vi "To Angle.vi"(1 "Reset":bool, 2 "Tolerance":dbl=1.0 format="%#_13g", 3 "Min. Power":dbl=0.1 format="%#_13g", 4 "Destination Angle":dbl) -> (0 "Power Change":dbl)   [LabVIEW 2014]
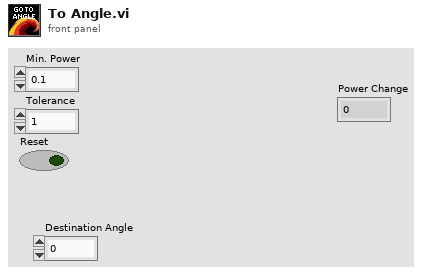
[diagram p1: front panel]
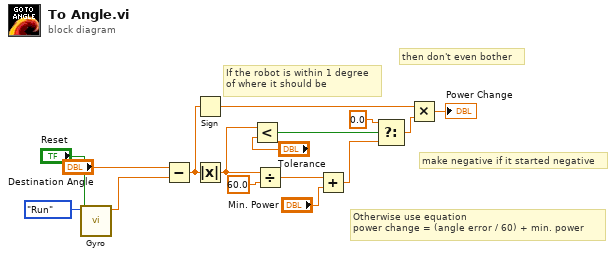
[diagram p0: block diagram]
diagram:
  # "make negative if it started negative"
  # "Otherwise use equation\npower change = (angle error / 60) + min. power"
  # "then don't even bother"
  # "If the robot is within 1 degree\nof where it should be"
  n1 = call "Gyro.vi"("Reset"="Reset", "Enum"=enum16{"Start", "Run", "End"}."Run") -> ("Angle"=w3:dbl)  [unwired: 9 in]
  n2 = Subtract(x="Destination Angle", y=w3) -> (x-y=w4:dbl)
  n3 = Sign(1:w4) -> (0:w9:dbl)
  n4 = Absolute Value(x=w4) -> (abs(x)=w8:dbl)
  n5 = Less?(x=w8, y="Tolerance") -> (x < y?=w6:bool)
  n6 = Divide(x=w8, y=60.0) -> (x/y=w11:dbl)
  n7 = Add(x=w11, y="Min. Power") -> (x+y=w12:dbl)
  n8 = Select(t=0.0, s=w6, f=w12) -> (s? t:f=w10:dbl)
  n9 = Multiply(x=w9, y=w10) -> (x*y=→"Power Change":dbl)
